vi "Configure Offset Modes.vi"(8 "error in (no error)":errorcluster, 10 "modes":u16[](array[ring]) items=["off", "on", "auto", "zero"], 11 "VGC in":refnum<class "PL Inficon VGC.lvclass">) -> (0 "error out":errorcluster, 2 "modes":u16[](array[ring]) items=["off", "on", "auto", "zero"], 3 "VGC out":refnum<class "PL Inficon VGC.lvclass">)   [LabVIEW 2015, in "PL Inficon VGC.lvclass"]
doc: "Configures offset modes."
uses:
  PL Inficon VGC.lvclass
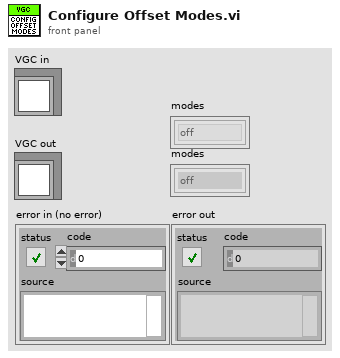
[diagram p1: front panel]
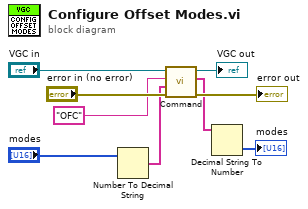
[diagram p0: block diagram]
diagram:
  n1 = Number To Decimal String(number="modes") -> (decimal integer string=w1:string[])  [unwired: 1 in]
  n2 = call "Command.vi"("error in (no error)"="error in (no error)", "parameters"=w1, "command"="OFC" ("format string"), "VGC in"="VGC in") -> ("error out"=→"error out":errorcluster, "response data"=w5:string[], "VGC out"=→"VGC out":refnum<class "PL Inficon VGC.lvclass">)  [unwired: 5 in]
  n3 = Decimal String To Number(string=w5) -> (number=→"modes":i32[])  [unwired: 2 in, 1 out]
